vi "Two Character Display Extension.vi"() -> ()   [LabVIEW 2014]
uses:
  <vilib>/myRIO/Instrument Drivers/Onboard IO/DIO/typedefs/DIO Reference.ctl
  <vilib>/myRIO/Common/Instrument Driver Framework/Utilities/typedefs/myRIO Generic Hardware Reference.ctl
  <vilib>/myRIO/Common/Instrument Driver Framework/Utilities/typedefs/Hardware Version Enum.ctl
  <vilib>/myRIO/Common/Instrument Driver Framework/Utilities/typedefs/myRIO v1.0 Reference.ctl
  <vilib>/myRIO/Common/Instrument Driver Framework/Utilities/typedefs/Generic FPGA Reference.ctl
  <vilib>/myRIO/Common/Instrument Driver Framework/myRIO v1.0/DIO/typedefs/DIO Channels List.ctl
  <vilib>/myRIO/Common/Instrument Driver Framework/myRIO v1.0/DIO/typedefs/DIO Channels Enum.ctl
  <vilib>/userdefined/High Color/nirio_resource_hc.ctl
  <vilib>/myRIO/Common/Instrument Driver Framework/Utilities/vis/Is FPGA Ref Available.vi
  <vilib>/myRIO/Common/Instrument Driver Framework/myRIO v1.0/DIO/vis/myRIO v1.1 Open DIO.vi
  <vilib>/myRIO/Instrument Drivers/Onboard IO/DIO/vis/Write.vi
  <vilib>/myRIO/Common/Instrument Driver Framework/Utilities/vis/Validate Channels.vi
  <vilib>/myRIO/Common/Instrument Driver Framework/myRIO v1.0/DIO/vis/myRIO v1.0 Reserve DIO.vi
  <vilib>/myRIO/Common/Instrument Driver Framework/myRIO v1.0/Resource Manager/vis/myRIO v1.0 Reserve Channel List.vi
  <vilib>/myRIO/Common/Instrument Driver Framework/myRIO v1.0/DIO/vis/myRIO v1.0 Build MUX Configuration DIO.vi
  <vilib>/myRIO/Common/Instrument Driver Framework/myRIO v1.0/Resource Manager/vis/myRIO v1.0 Reserve Channel.vi
  <vilib>/myRIO/Common/Instrument Driver Framework/myRIO v1.0/Resource Manager/vis/myRIO v1.0 Unreserve Channel.vi
  <vilib>/myRIO/Common/Instrument Driver Framework/myRIO v1.0/Resource Manager/vis/myRIO v1.0 Create Configuration List.vi
  <vilib>/myRIO/Common/Instrument Driver Framework/myRIO v1.0/Resource Manager/vis/myRIO v1.0 Build Mutex Name.vi
  <vilib>/Utility/VariantDataType/GetNumericInfo.vi
  <vilib>/Utility/error.llb/Error Cluster From Error Code.vi
  <vilib>/myRIO/Common/Instrument Driver Framework/myRIO v1.0/myRIO v1.1 Open.vi
  <vilib>/myRIO/Common/Instrument Driver Framework/Utilities/vis/IO Manager.vi
  <vilib>/myRIO/Common/Instrument Driver Framework/Utilities/vis/Configuration Manager.vi
  <vilib>/myRIO/Common/Instrument Driver Framework/myRIO v1.0/Resource Manager/vis/myRIO v1.0 Configure IO.vi
  <vilib>/myRIO/Common/Instrument Driver Framework/myRIO v1.0/myRIO v1.0 Close.vi
  <vilib>/myRIO/Common/Instrument Driver Framework/myRIO v1.0/DIO/vis/myRIO v1.0 Write DIO.vi
  <vilib>/myRIO/Express VI/Onboard IO/DO/DO Express VI.xnode
  <vilib>/myRIO/Instrument Drivers/Onboard IO/DIO/vis/myRIO DIO Open.xnode
  <vilib>/myRIO/Instrument Drivers/Onboard IO/DIO/DIO.lvlib
panel:
  in  "Alarm M1":bool[](array[boolean])
  in  "Alarm M10":bool[](array[boolean])
  in  "Alarm S10":bool[](array[boolean])
  in  "Alarm S1":bool[](array[boolean])
  out "Current Time":timestamp
  out "M1":bool[](array[boolean])
  out "M10":bool[](array[boolean])
  out "S10":bool[](array[boolean])
  out "S1":bool[](array[boolean])
  in  "Stop Button":bool
  # "Set Alarm"
  # "Minutes"
  # "Seconds"
  # "Minutes"
  # "Seconds"
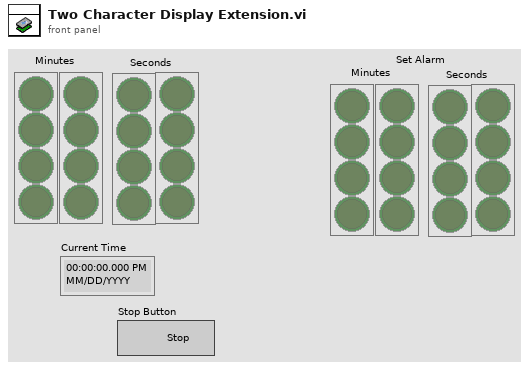
[diagram p1: front panel]
types:
  T1 = typedef "DIO.lvlib/DIO Reference.ctl" = cluster{"myRIO Reference":T2, "DIO Channels List":T6}
  T2 = typedef "myRIO Generic Hardware Reference.ctl" = cluster{"myRIO Model":T3, "myRIO Hardware Reference":T4}
  T3 = typedef "Hardware Version Enum.ctl" = enum16{"Unknown", "myRIO-1900", "myRIO-1950"}
  T4 = typedef "myRIO v1.0 Reference.ctl" = cluster{"Generic FPGA Reference":T5, "Allow multiple opens":bool}
  T5 = typedef "Generic FPGA Reference.ctl" = refnum<k20>
  T6 = typedef "DIO Channels List.ctl" = T7[]
  T7 = typedef "DIO Channels Enum.ctl" = enum16{"Not Connected", "C/DIO0", "C/DIO1", "C/DIO2", "C/DIO3", "C/DIO4", "C/DIO5", "C/DIO6", "C/DIO7", "A/DIO0", "A/DIO1", "A/DIO2", "A/DIO3", "A/DIO4", "A/DIO5", "A/DIO6", "A/DIO7", "A/DIO8", "A/DIO9", "A/DIO10", "A/DIO11", "A/DIO12", "A/DIO13", "A/DIO14", "A/DIO15", "B/DIO0", "B/DIO1", "B/DIO2", "B/DIO3", "B/DIO4", "B/DIO5", "B/DIO6", "B/DIO7", "B/DIO8", "B/DIO9", "B/DIO10", "B/DIO11", "B/DIO12", "B/DIO13", "B/DIO14", "B/DIO15", "LED0", "LED1", "LED2", "LED3", "Button0"}
  T8 = typedef "nirio_resource_hc.ctl" = tag
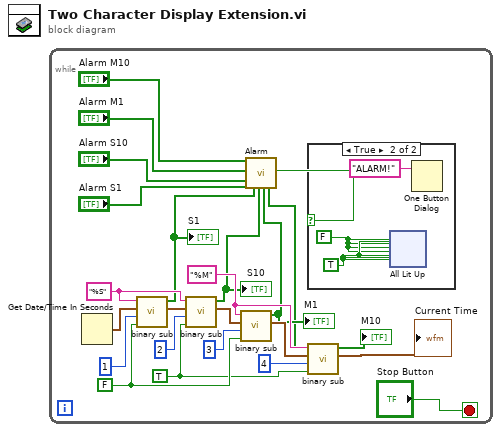
[diagram p0: block diagram]
diagram:
  n1 = while {
    stop <- "Stop Button" stop-if-true
    w11 = "%M" ("time format string (%c)")
    w17 = TRUE ("Tens?")
    w18 = FALSE ("Tens?")
    w10 = "%S" ("time format string (%c)")
    n2 = Get Date/Time In Seconds() -> (seconds since 1Jan1904=w12:timestamp)
    n3 = call "binary sub.vi"("Tens?"=w18, "order"=u8 1, "Time Stamp"=w12, "time format string (%c)"=w10) -> ("Time Stamp 2"=w21:timestamp, "Array"=w9:bool[])  [unwired: 6 in]
    "S1" <- w9
    n4 = call "binary sub.vi"("Tens?"=w17, "order"=u8 2, "Time Stamp"=w21, "time format string (%c)"=w10) -> ("Time Stamp 2"=w20:timestamp, "Array"=w8:bool[])  [unwired: 6 in]
    "S10" <- w8
    n5 = call "binary sub.vi"("Tens?"=w18, "order"=u8 3, "Time Stamp"=w20, "time format string (%c)"=w11) -> ("Time Stamp 2"=w19:timestamp, "Array"=w7:bool[])  [unwired: 6 in]
    "M1" <- w7
    n6 = call "binary sub.vi"("Tens?"=w17, "order"=u8 4, "Time Stamp"=w19, "time format string (%c)"=w11) -> ("Time Stamp 2"=→"Current Time":timestamp, "Array"=w6:bool[])  [unwired: 6 in]
    "M10" <- w6
    n7 = call "Alarm.vi"("Alarm M10"="Alarm M10", "Alarm M1"="Alarm M1", "Alarm S10"="Alarm S10", "Alarm S1"="Alarm S1", "Second Ones"=w9, "Second Tens"=w8, "Minute Ones"=w7, "Minute Tens"=w6) -> ("Alarm"=w1:bool)  [unwired: 11 in]
    n8 = case shown="True" w1 {
      frame False {
      }
      frame True {
        w25 = TRUE
        w24 = FALSE
        n9 = xnode "All Lit Up"("B/DIO0 (Pin 11)"=w24, "B/DIO1 (Pin 13)"=w24, "B/DIO2 (Pin 15)"=w24, "B/DIO3 (Pin 17)"=w24, "B/DIO4 (Pin 19)"=w25, "B/DIO5 (Pin 21)"=w25, "B/DIO6 (Pin 23)"=w25, "B/DIO7 (Pin 25)"=w25) -> ()  [unwired: 1 in, 1 out]
        n10 = One Button Dialog(message="ALARM!") -> ()  [unwired: 1 in, 1 out]
      }
    }
  }
